vi "Read Port Settings from JSON.vi"() -> (3 "Port settings":T1)   [LabVIEW 2020, in "GUI.lvlib" / "GUI.lvclass"]
uses:
  GUI.lvclass
  Modbus/Modbus/Port Settings.ctl
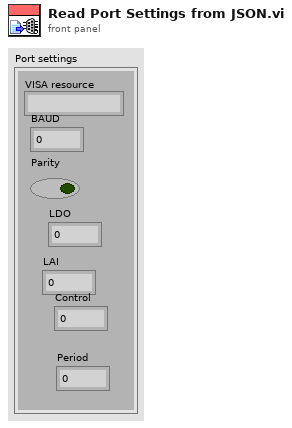
[diagram p1: front panel]
types:
  T1 = typedef "Port Settings.ctl" = cluster{"VISA resource":string, "BAUD":u16, "Parity":bool, "LDO":u16, "LAI":u16, "Control":u16, "Period":u16}
  T2 = enum16{"open", "replace", "create", "open or create", "replace or create", "replace or create with confirmation"}
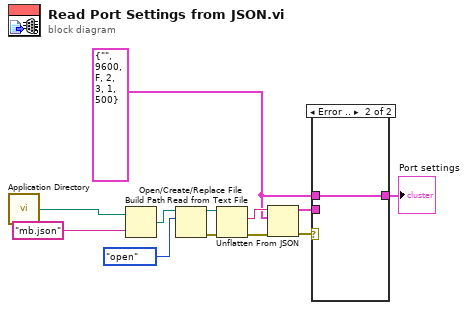
[diagram p0: block diagram]
diagram:
  w2 = T1 {"VISA resource"="", "BAUD"=9600, "Parity"=FALSE, "LDO"=2, "LAI"=3, "Control"=1, "Period"=500} ("Port settings")
  n1 = call <vilib>:"Application Directory.vi"() -> ("Application Directory"=w12:path)
  n2 = Build Path(base path=w12, name or relative path="mb.json") -> (appended path=w10:path)
  n3 = Open/Create/Replace File(file path (use dialog)=w10, operation (0:open)=T2."open") -> (refnum out=w6:refnum<file>, error out=w5:errorcluster)  [unwired: 4 in, 1 out]
  n4 = Read from Text File(file (use dialog)=w6, error in=w5) -> (text=w7:string, error out=w8:errorcluster)  [unwired: 2 in, 2 out]
  n5 = Unflatten From JSON(JSON string=w7, type and defaults=w2, error in (no error)=w8) -> (value=w3:T1, error out=w4:errorcluster)  [unwired: 4 in]
  n6 = case shown="Error .." w4 {
    tunnel: w3 -> [w13 _]
    tunnel: w2 -> [_ w14]
    tunnel: [w13 w14] -> w1
    frame No Error {
    }
    frame Error {
    }
  }
  "Port settings" <- w1
